vi "StartSession.vi"(0 "device Address":string, 1 "bitfile Path":string) -> (19 "Error Out":errorcluster)   [LabVIEW 2015]
doc: "Configures device parameters for an NI 5170/5171"
uses:
  <instrlib>/HSAI-RIO/Types/v1/Host/Typedefs/Reference Clock Source.ctl
  OscopeAPI/Device Session.lvclass
  <instrlib>/HSAI-RIO/Types/v1/Host/niHSAI Types v1 Host.lvlib
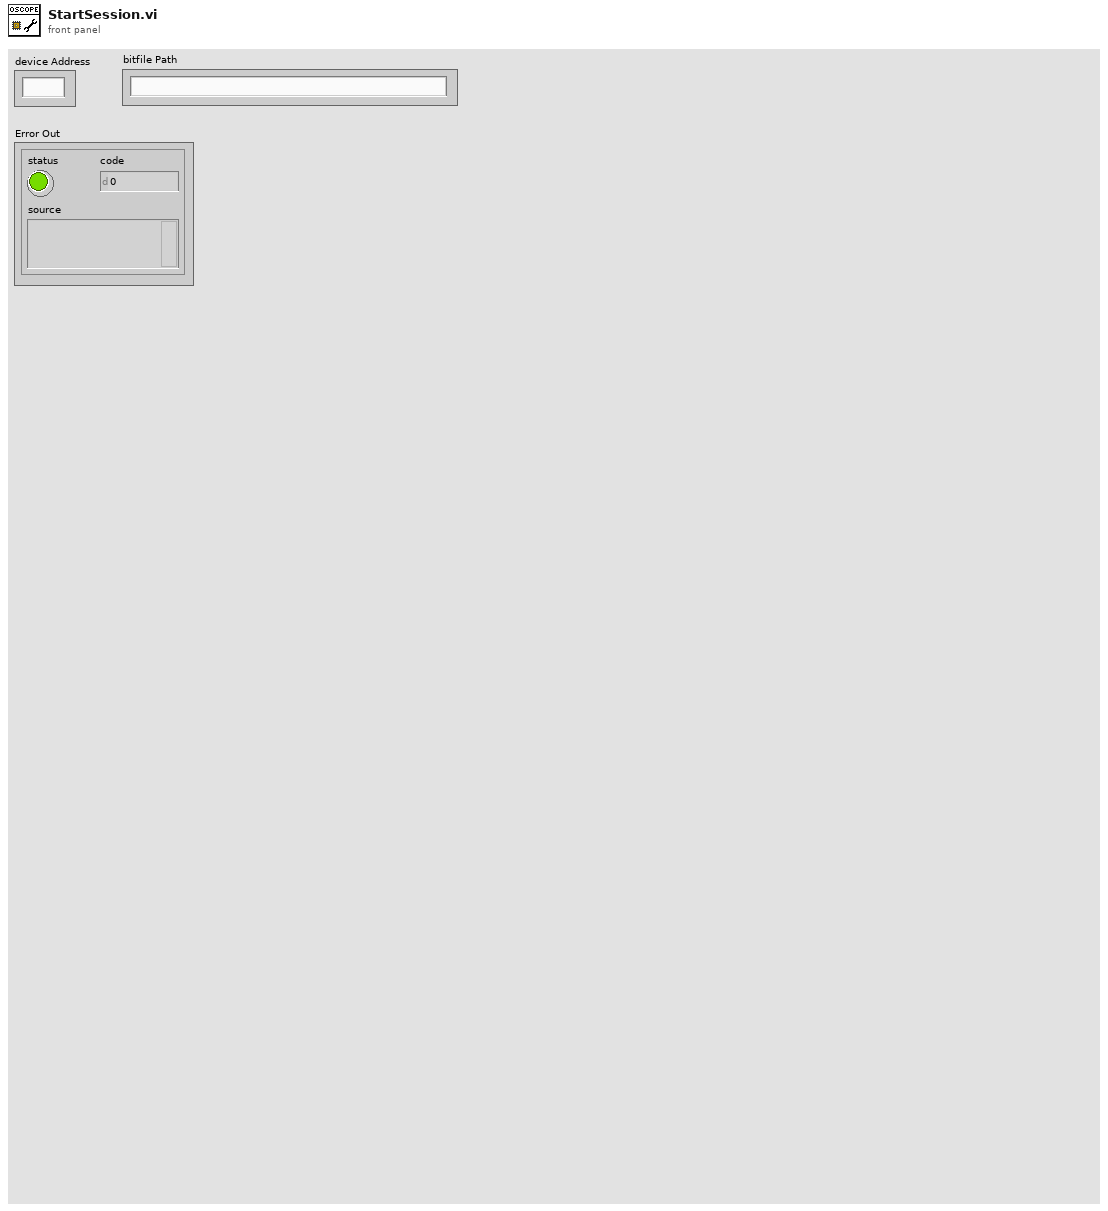
[diagram p1: front panel]
types:
  T1 = typedef "niHSAI Types v1 Host.lvlib/Reference Clock Source.ctl" = enum8{"None", "Clock In", "PXI Clock"}
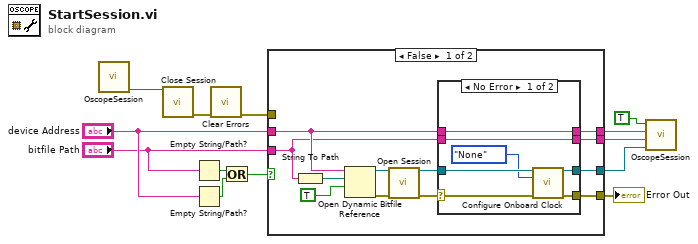
[diagram p0: block diagram]
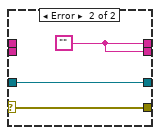
[diagram p2: hidden frame]
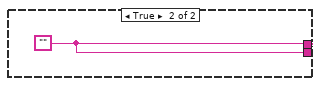
[diagram p3: hidden frame]
diagram:
  n1 = call "OscopeSession.vi"() -> ("Session Out"=w3:refnum<class "Device Session.lvclass">)  [unwired: 9 in, 2 out]
  n2 = call "Close Session.vi"("device session in"=w3) -> ("error out"=w2:errorcluster)  [unwired: 14 in]
  n3 = Empty String/Path?(string/path="bitfile Path") -> (empty?=w9:bool)
  n4 = Empty String/Path?(string/path="device Address") -> (empty?=w10:bool)
  n5 = call <vilib>:"Clear Errors.vi"("error in (no error)"=w2) -> ("error out"=w1:errorcluster)  [unwired: 5 in, 1 out]
  n6 = Or(x=w9, y=w10) -> (x .or. y?=w13:bool)
  n7 = case shown="False" w13 {
    tunnel: "device Address" -> [w16 _]
    tunnel: "bitfile Path" -> [w14 _]
    tunnel: [w17 w36] -> w7
    tunnel: [w15 w36] -> w6
    tunnel: [w19 _] -> w5
    tunnel: [w20 _] -> w4
    tunnel: w1 -> [_ _]
    frame False {
      n8 = String To Path(string=w14) -> (path=w24:path)
      n9 = Open Dynamic Bitfile Reference(0:w16, 1:w24, 2:TRUE ("Run When Loaded")) -> (5:w22:refnum<k20>, 8:w25:errorcluster)  [unwired: 2 in]
      n10 = call "Open Session.vi"("fpga in"=w22, "error in"=w25) -> ("device session out"=w18:refnum<class "Device Session.lvclass">, "error out"=w21:errorcluster)  [unwired: 12 in]
      n11 = case shown="No Error" w21 {
        selector: w21 -> [w30 w35]
        tunnel: [w29 w35] -> w20
        tunnel: [w27 w34] -> w19
        tunnel: w18 -> [w28 w34]
        tunnel: [w32 w33] -> w17
        tunnel: w16 -> [w32 _]
        tunnel: [w31 w33] -> w15
        tunnel: w14 -> [w31 _]
        frame No Error {
          n12 = call "Configure Onboard Clock.vi"("device session in"=w28, "reference clock source"=Reference_Clock_Source."None", "error in"=w30) -> ("device session out"=w27:refnum<class "Device Session.lvclass">, "error out"=w29:errorcluster)  [unwired: 9 in, 2 out]
        }
        frame Error {
          w33 = ""
        }
      }
    }
    frame True {
      w36 = ""
    }
  }
  "Error Out" <- w4
  n13 = call "OscopeSession.vi"("Session In"=w5, "Bitfile Path In"=w6, "Device Address In"=w7, "Write"=TRUE) -> ()  [unwired: 5 in, 3 out]
